vi "Hold Robot.vi"(11 "Reset Encoders?":bool) -> (3 "Speed Output":cluster{"output":dbl, "output":dbl})   [LabVIEW 2011]
uses:
  <vilib>/addons/control/pid/pid.llb/PID (DBL).vi
  <vilib>/addons/control/pid/NI_PID_pid.lvlib
panel:
  out "Right Error":dbl(graph)
  out "Left Error":dbl(graph)
  in  "PID gains":T1={"proportional gain (Kc)"=1.0, "integral time (Ti, min)"=0.01, "derivative time (Td, min)"=0.0} {"derivative time (Td, min)" format="%.3f"; "integral time (Ti, min)" format="%.3f"; "proportional gain (Kc)" format="%.3f"}
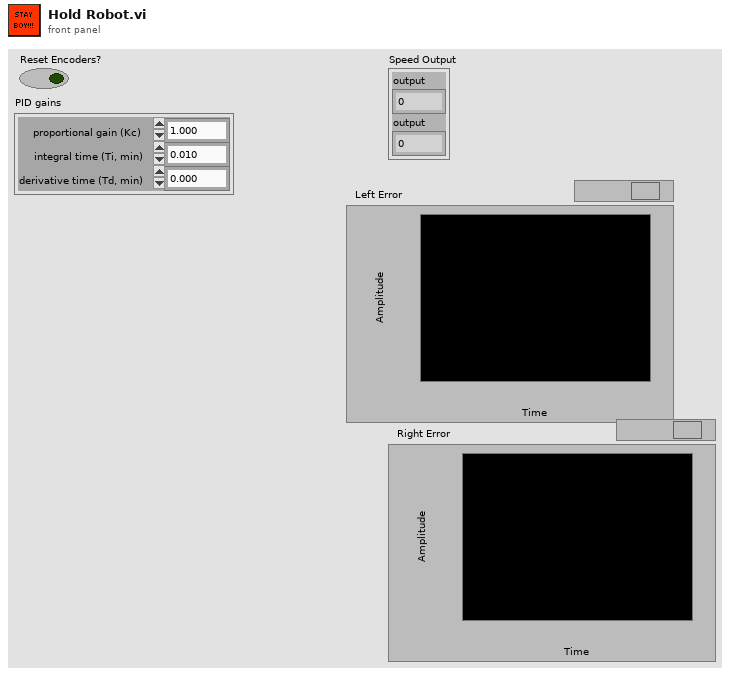
[diagram p1: front panel]
types:
  T1 = cluster{"proportional gain (Kc)":dbl, "integral time (Ti, min)":dbl, "derivative time (Td, min)":dbl}
  T2 = cluster{"Speed Right":dbl, "Distance Right":dbl, "Speed Left":dbl, "Distance Left":dbl}
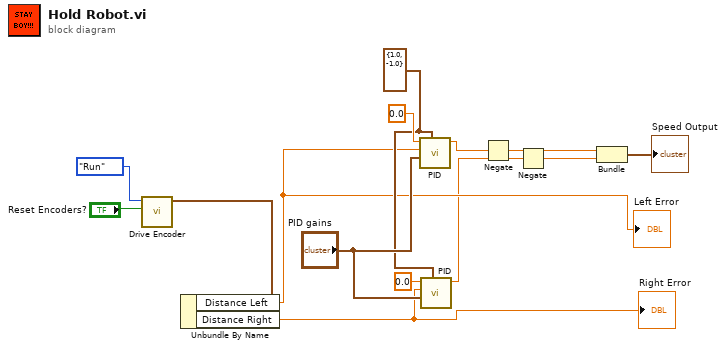
[diagram p0: block diagram]
diagram:
  w7 = cluster{"output high":dbl, "output low":dbl} {"output high"=1.0, "output low"=-1.0} ("output range")
  n1 = call "Drive Encoder.vi"("Reset"="Reset Encoders?", "Enum"=enum16{"Init", "Run", "End"}."Run" ("Mode")) -> ("Encoder Values"=w10:T2)  [unwired: 9 in]
  n2 = Unbundle By Name(w10) -> ("Distance Left"=w5:dbl, "Distance Right"=w6:dbl)
  "Left Error" <- w5
  "Right Error" <- w6
  n3 = call-poly <vilib>:"PID.vi"("output range"=w7, "PID gains"="PID gains", "process variable"=w5, "setpoint"=0.0) -> ("output"=w3:dbl)  [unwired: 6 in, 1 out]
  n4 = call-poly <vilib>:"PID.vi"("output range"=w7, "PID gains"="PID gains", "process variable"=w6, "setpoint"=0.0) -> ("output"=w4:dbl)  [unwired: 6 in, 1 out]
  n5 = Negate(x=w3) -> (-x=w2:dbl)
  n6 = Negate(x=w4) -> (-x=w1:dbl)
  n7 = Bundle(w2, w1) -> (→"Speed Output":cluster{dbl, dbl})  [unwired: 1 in]
